vi "temp setpoint(SubVI).vi"(0 "Temperature 2":dbl=300.0, 1 "Temperature":dbl=300.0, 3 "Rate":dbl=10.0, 4 "Instrument Ref":refnum<k24>, 5 "ch str":string, 6 "Delay":dbl, 9 "steps number":i32, 11 "Approach":i32(ring) items=["FastSettle", "NoOvershoot"], 12 "data":refnum<queue>, 13 "config":refnum<queue>, 14 "Resource In":refnum<visa-resource-name>) -> (10 "错误输出":errorcluster)   [LabVIEW 2019, in "SubVI.lvlib"]
uses:
  SubVI.lvlib
  lib/QDInstrument.dll
  config.ctl
panel:
  # "(真是通道1，假是通道2)"
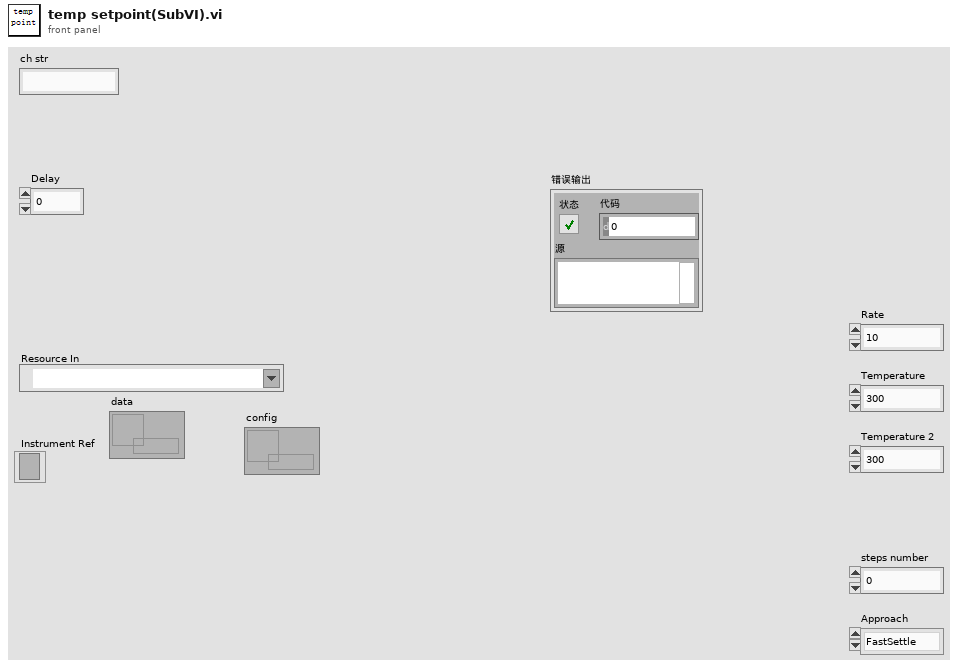
[diagram p1: front panel]
types:
  T1 = typedef "config.ctl" = cluster{"error":bool, "initialize":string, "数值":dbl, "6221":cluster{"6221 Resource":refnum<visa-resource-name>, "Delta status":bool}, "7001":cluster{"Ch":bool}}
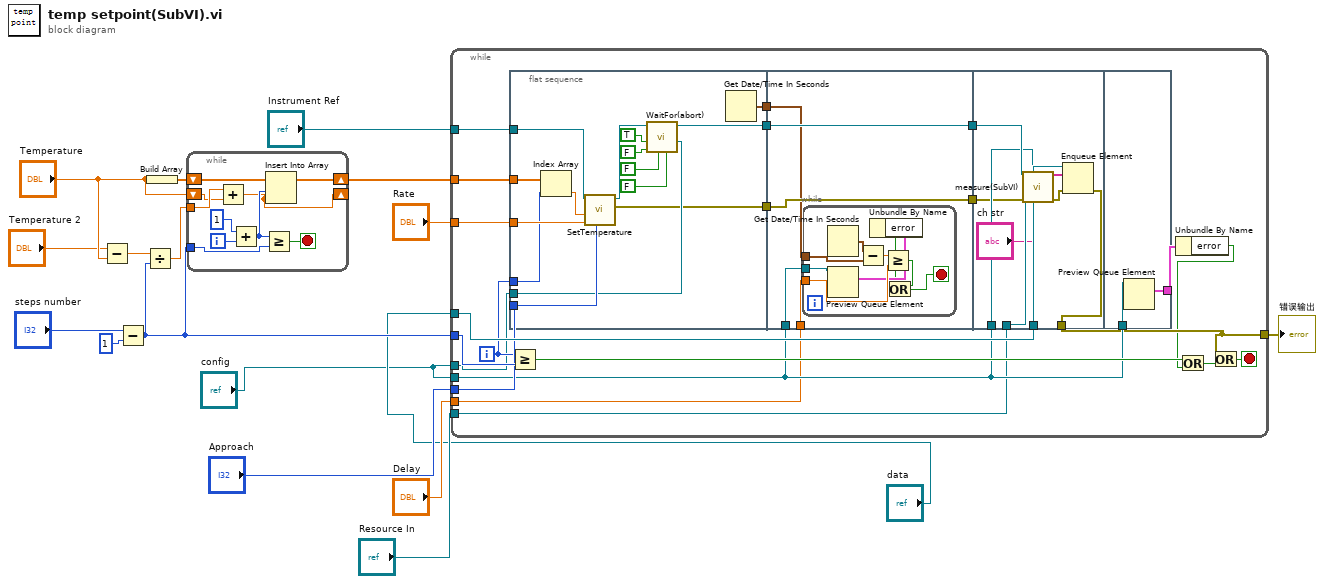
[diagram p0: block diagram]
diagram:
  n1 = Subtract(x="Temperature 2", y="Temperature") -> (x-y=w14:dbl)
  n2 = Subtract(x="steps number", y=1) -> (x-y=w4:i32)
  n3 = Divide(x=w14, y=w4) -> (x/y=w16:dbl)
  n4 = Build Array("Temperature") -> (w15:dbl[])
  n5 = while {
    shift-right: [w27] -> w10
    shift-left: w15 -> [w26]
    tunnel: w16 -> [w21]
    tunnel: w4 -> [w20]
    shift-right: [w19] -> _
    shift-left: "Temperature" -> [w18]
    i -> [w25]
    stop <- w22 stop-if-true
    n6 = Add(x=w21, y=w18) -> (x+y=w19:dbl)
    n7 = Add(x=1, y=w25) -> (x+y=w23:i32)
    n8 = Greater Or Equal?(x=w23, y=w20) -> (x >= y?=w22:bool)
    n9 = Insert Into Array(array=w26, index=w23, new element=w19) -> (w27:dbl[])
  }
  n10 = while {
    tunnel: w4 -> [w47]
    tunnel: "data" -> [w49]
    tunnel: "config" -> [w34]
    tunnel: "Approach" -> [w46]
    tunnel: "Rate" -> [w45]
    tunnel: "Instrument Ref" -> [w44]
    tunnel: w10 -> [w43]
    tunnel: "config" -> [w41]
    tunnel: [w30] -> w8
    tunnel: "Delay" -> [w33]
    tunnel: "Resource In" -> [w31]
    i -> [w42]
    stop <- w39 stop-if-true
    n11 = flat-sequence {
      tunnel: [w53] -> w38
      tunnel: w46 -> [w62]
      tunnel: w45 -> [w61]
      tunnel: w44 -> [w60]
      tunnel: w43 -> [w59]
      tunnel: w42 -> [w58]
      tunnel: w41 -> [w52]
      tunnel: [w51] -> w36
      tunnel: [w50] -> w32
      tunnel: w38 -> [w69]
      tunnel: [w69] -> w37
      tunnel: w36 -> [w68]
      tunnel: [w68] -> w35
      tunnel: w34 -> [w67]
      tunnel: w33 -> [w66]
      tunnel: w32 -> [w65]
      tunnel: w37 -> [w86]
      tunnel: w49 -> [w87]
      tunnel: w34 -> [w85]
      tunnel: w35 -> [w83]
      tunnel: w31 -> [w82]
      tunnel: [w80] -> w30
      tunnel: w34 -> [w89]
      tunnel: [w88] -> w29
      frame #0 {
        n12 = Index Array(array=w59, index=w58) -> (element=w64:dbl)
        n13 = call "SetTemperature.vi"("Approach"=w62, "Rate"=w61, "Temperature"=w64, "Instrument Ref In"=w60) -> ("error out"=w51:errorcluster, "Instrument Ref Out"=w63:refnum<k24>)  [unwired: 3 in, 1 out]
        n14 = call "WaitFor(abort).vi"("config"=w52, "Wait For Chamber"=FALSE, "Wait For Position"=FALSE, "Wait For Field"=FALSE, "Wait For Temperature"=TRUE, "Instrument Ref In"=w63) -> ("Instrument Ref Out"=w53:refnum<k24>)  [unwired: 4 in, 1 out]
        n15 = Get Date/Time In Seconds() -> (seconds since 1Jan1904=w50:timestamp)
      }
      frame #1 {
        n16 = while {
          tunnel: w65 -> [w77]
          tunnel: w66 -> [w75]
          tunnel: w67 -> [w73]
          stop <- w70 stop-if-true
          n17 = Get Date/Time In Seconds() -> (seconds since 1Jan1904=w78:timestamp)
          n18 = Preview Queue Element(queue=w73) -> (element=w72:T1)  [unwired: 2 in, 3 out]
          n19 = Subtract(x=w78, y=w77) -> (x-y=w76:dbl)
          n20 = Unbundle By Name(w72) -> ("error"=w71:bool)
          n21 = Greater Or Equal?(x=w76, y=w75) -> (x >= y?=w74:bool)
          n22 = Or(x=w74, y=w71) -> (x .or. y?=w70:bool)
        }
      }
      frame #2 {
        n23 = call "measure(SubVI).vi"(".NET引用句柄输入"=w86, "config"=w85, 7:w82, "error in (no error)"=w83, "ch str"="ch str") -> ("data"=w84:string[], "error out"=w81:errorcluster)  [unwired: 9 in]
        n24 = Enqueue Element(queue=w87, element=w84, error in (no error)=w81) -> (error out=w80:errorcluster)  [unwired: 1 in, 2 out]
      }
      frame #3 {
        n25 = Preview Queue Element(queue=w89) -> (element=w88:T1)  [unwired: 2 in, 3 out]
      }
    }
    n26 = Greater Or Equal?(x=w42, y=w47) -> (x >= y?=w48:bool)
    n27 = Unbundle By Name(w29) -> ("error"=w28:bool)
    n28 = Or(x=w48, y=w28) -> (x .or. y?=w40:bool)
    n29 = Or(x=w30, y=w40) -> (x .or. y?=w39:bool)
  }
  "错误输出" <- w8
